vi "Sub Vi slope.vi"() -> ()   [LabVIEW 2020]
panel:
  out "Slope":dbl
  in  "X1":dbl
  in  "X2":dbl
  in  "Y2":dbl
  in  "Y1":dbl
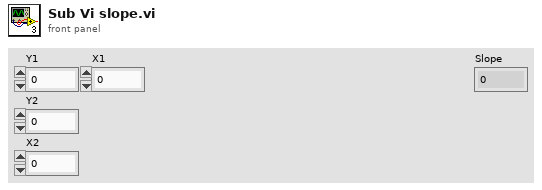
[diagram p1: front panel]
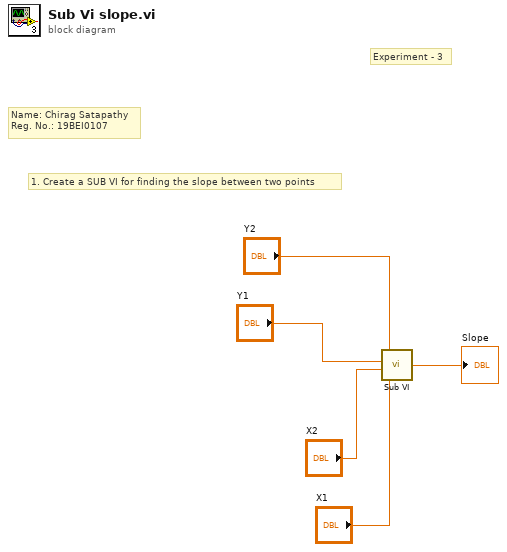
[diagram p0: block diagram]
diagram:
  # "Experiment - 3"
  # "1. Create a SUB VI for finding the slope between two points"
  # "Name: Chirag Satapathy\nReg. No.: 19BEI0107"
  n1 = call "Sub VI.vi"("X1"="X1", "X2"="X2", "Y1"="Y1", "Y2"="Y2") -> ("Slope"=→"Slope":dbl)
